vi "Climber.vi"   [LabVIEW 2016]
uses:
  <vilib>/Rock Robotics/WPI/Utilities/WPI_GetSetVariantRefNum.vi
types:
  T1 = typedef "WPI_JoystickDevRef.ctl" = cluster{"Device":T2}
  T2 = typedef "WPI_JoystickDeviceEnum.ctl" = enum16{"USB 0", "USB 1", "USB 2", "USB 3", "USB 4", "USB 5"}
  T3 = typedef "WPI_MotorControlDeviceRef.ctl" = cluster{"DeviceStatus":errorcluster, "Type":T4, "PWM":cluster{"PWM Channel":T5, "DeadBand":T6}, "CAN":cluster{"Device Number":u8, "SetOutput VI Ref":variant, "GetOutput VI Ref":variant, "Enable VI Ref":variant, "Disable VI Ref":variant, "Data":variant}, "Invert":bool}
  T4 = typedef "WPI_MotorControlType.ctl" = enum16{"PWM", "CAN"}
  T5 = typedef "FPGA_DIOPWMChannel.ctl" = enum8{"PWM 0", "PWM 1", "PWM 2", "PWM 3", "PWM 4", "PWM 5", "PWM 6", "PWM 7", "PWM 8", "PWM 9", "PWM MXP 0", "PWM MXP 1", "PWM MXP 2", "PWM MXP 3", "PWM MXP 4", "PWM MXP 5", "PWM MXP 6", "PWM MXP 7", "PWM MXP 8", "PWM MXP 9", "Invalid"}
  T6 = typedef "WPI_PWMDeadband.ctl" = cluster{"Name":string, "maxPositivePwm":i32, "minPositivePwm":i32, "centerPwm":i32, "maxNegativePwm":i32, "minNegativePwm":i32, "angularRange":u16}
  T7 = typedef "WPI_ServoDeviceRef.ctl" = cluster{"DeviceStatus":errorcluster, "PWM Channel":T5, "DeadBand":T6}
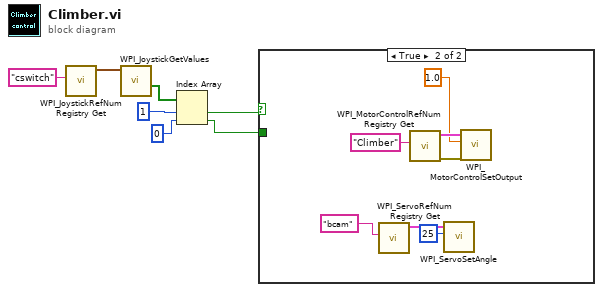
[diagram p0: block diagram]
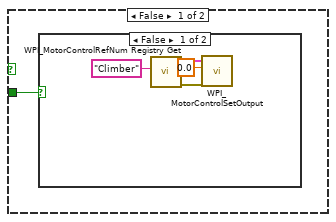
[diagram p2: hidden frame]
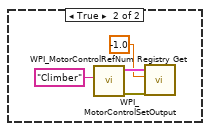
[diagram p3: hidden frame]
diagram:
  n1 = call <vilib>:"WPI_JoystickRefNum Registry Get.vi"("refnum name"="cswitch") -> ("JoystickDevRef"=w7:T1)  [unwired: 9 in, 1 out]
  n2 = call <vilib>:"WPI_JoystickGetValues.vi"("JoystickDevRef"=w7) -> ("Buttons"=w6:bool[])  [unwired: 6 in, 4 out]
  n3 = Index Array(array=w6, index #1=1 ("index"), index #2=0 ("index")) -> (element #1=w1:bool, element #2=w2:bool)
  n4 = case shown="True" w1 {
    tunnel: w2 -> [w8 _]
    frame False {
      n5 = case shown="False" w8 {
        frame False {
          n6 = call <vilib>:"WPI_MotorControlRefNum Registry Get.vi"("refnum name"="Climber") -> ("error out"=w11:errorcluster, "MotorControlDevRef"=w10:T3)  [unwired: 9 in]
          n7 = call <vilib>:"WPI_MotorControlSetOutput.vi"("error in (no error)"=w11, "Output"=0.0, "MotorControlDevRef"=w10) -> ()  [unwired: 6 in, 3 out]
        }
        frame True {
          n8 = call <vilib>:"WPI_MotorControlRefNum Registry Get.vi"("refnum name"="Climber") -> ("error out"=w15:errorcluster, "MotorControlDevRef"=w16:T3)  [unwired: 9 in]
          n9 = call <vilib>:"WPI_MotorControlSetOutput.vi"("error in (no error)"=w15, "Output"=-1.0, "MotorControlDevRef"=w16) -> ()  [unwired: 6 in, 3 out]
        }
      }
    }
    frame True {
      n10 = call <vilib>:"WPI_ServoRefNum Registry Get.vi"("refnum name"="bcam") -> ("ServoDeviceRef"=w18:T7)  [unwired: 9 in, 1 out]
      n11 = call <vilib>:"WPI_MotorControlRefNum Registry Get.vi"("refnum name"="Climber") -> ("error out"=w22:errorcluster, "MotorControlDevRef"=w23:T3)  [unwired: 9 in]
      n12 = call <vilib>:"WPI_ServoSetAngle.vi"("Angle"=25, "ServoDeviceRef"=w18) -> ()  [unwired: 8 in, 2 out]
      n13 = call <vilib>:"WPI_MotorControlSetOutput.vi"("error in (no error)"=w22, "Output"=1.0, "MotorControlDevRef"=w23) -> ()  [unwired: 6 in, 3 out]
    }
  }
